vi "Kinesis - BNT - Connect.vi"() -> ()   [LabVIEW 2015]
doc: "Shows how to set and get the NanoTrak circle home position."
uses:
  C:/Users/fmovagharnemati/OneDrive - THORLABS Inc/Desktop/Kinesis_with_LabVIEW_Examples_LV12 - v3/Thorlabs.MotionControl.Controls.dll
  Thorlabs.MotionControl.Controls.dll
panel:
  in  "?":bool
  in  "SerialNumber":string
  in  "BenchtopNanoTrakControl":refnum<k24>(container)
  # "Notes:"
  # "- Ensure that the appropriate .DLLs are copied into your Project Folder. Check that the correct bit type are used depending on your version of LabVIEW\ni.e. 32-bit or 64-bit.\n\n\n\n\n\n\n\n\n\n\n\n\n\n\n- Open the example VI through the LabVIEW Project Explorer to correctly load the User Interface from Thorlabs.MotionControl.Controls.dll."
  # "Thorlabs Hardware: BNT001/IR\nhttps://www.thorlabs.com/newgrouppage9.cfm?objectgroup_id=1194&pn=BNT001/IR"
  # "Description: This VI will enable you to connect to & safely disconnect to a BNT001 device."
  # "Instructions: \n1) Connect your BNT001 device to your PC & power the device. For full device setup, the device product manual can be found on our website here.\n - https://www.thorlabs.com/thorproduct.cfm?partnumber=BNT001/IR\n2) Enter the device serial number below.\n3) Click 'Run' in the LabVIEW Toolbar.\n4) To end the Program, click 'END'."
  # "Example Image of .NET Controller - VI opened via Project Explorer/ not opened via Project Explorer"
  # "VI Not Opened via Project Explorer"
  # "VI Opened via Project Explorer"
  # "- To explore the range of methods available, please visit the .NET API, included with your Kinesis software.\n\n- For tips on building your own VIs with Thorlabs Motion Control Hardware, please see our LabVIEW Guide here.\nhttps://www.thorlabs.com/newgrouppage9.cfm?objectgroup_id=10285"
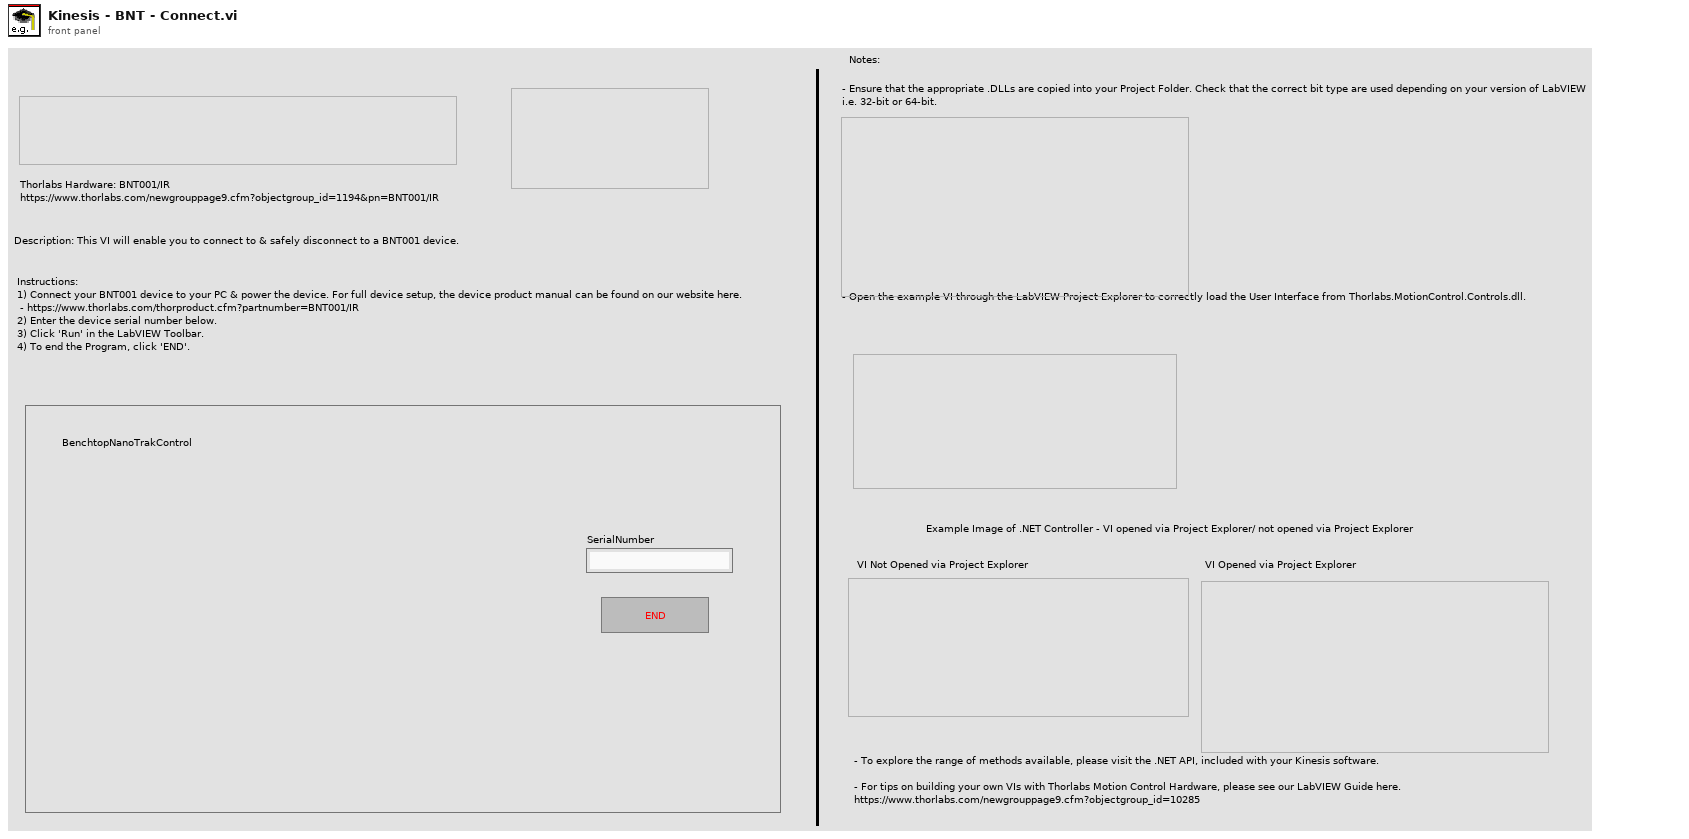
[diagram p1: front panel]
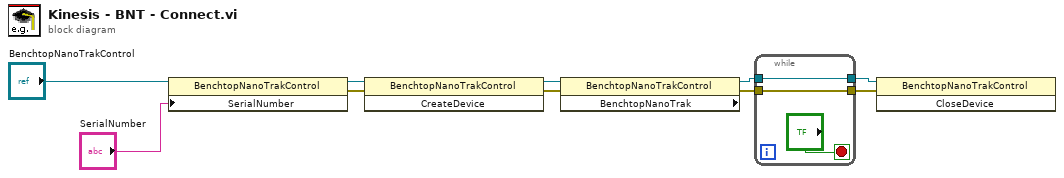
[diagram p0: block diagram]
diagram:
  n1 = property class="BenchtopNanoTrakControl"(reference="BenchtopNanoTrakControl", "SerialNumber"="SerialNumber") -> (reference out=w8:refnum<k24>, error out=w5:errorcluster)  [unwired: 1 in]
  n2 = invoke class="BenchtopNanoTrakControl" method="CreateDevice"(reference=w8, error in=w5) -> (reference out=w7:refnum<k24>, error out=w6:errorcluster)  [unwired: 1 in, 1 out]
  n3 = property class="BenchtopNanoTrakControl" props=["BenchtopNanoTrak"](reference=w7, error in=w6) -> (reference out=w1:refnum<k24>, error out=w3:errorcluster)  [unwired: 1 out]
  n4 = while {
    tunnel: [w12] -> w4
    tunnel: w3 -> [w12]
    tunnel: [w11] -> w2
    tunnel: w1 -> [w11]
    stop <- "?" stop-if-true
  }
  n5 = invoke class="BenchtopNanoTrakControl" method="CloseDevice"(reference=w2, error in=w4) -> ()  [unwired: 1 in, 3 out]
